vi "Spectrum Merge Wavelengths v10.5.0.vi"(2 "Wavelengths (nm)":dbl[](array[numeric]), 3 "Raw Spectrum":dbl[](array[numeric])) -> (0 "Spectrum-Array":dbl[][](array[numeric]), 1 "Spectrum-Cluster":T1(array[cluster]))   [LabVIEW 2010]
panel:
  out "Ausgangs-Cluster":T2
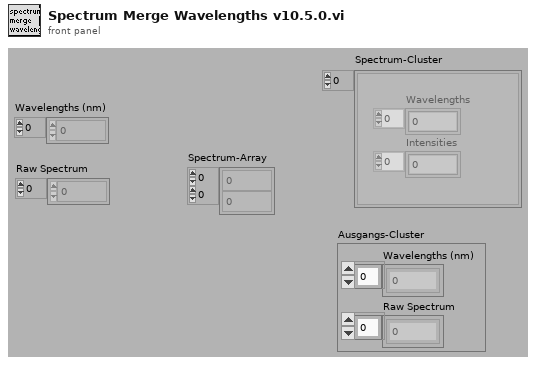
[diagram p1: front panel]
types:
  T1 = cluster{"Intensities":dbl[], "Wavelengths":dbl[]}[]
  T2 = cluster{"Wavelengths (nm)":dbl[], "Raw Spectrum":dbl[]}
  T3 = cluster{"Wavelengths (nm)":dbl[], "Raw Spectrum":dbl[]}[]
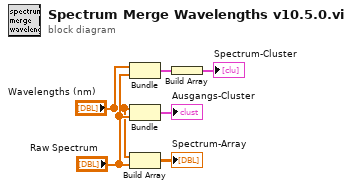
[diagram p0: block diagram]
diagram:
  n1 = Bundle("Wavelengths (nm)"="Wavelengths (nm)", "Raw Spectrum"="Raw Spectrum") -> (w4:T2)  [unwired: 1 in]
  n2 = Bundle("Wavelengths (nm)"="Wavelengths (nm)", "Raw Spectrum"="Raw Spectrum") -> (→"Ausgangs-Cluster":T2)  [unwired: 1 in]
  n3 = Build Array("Wavelengths (nm)", "Raw Spectrum") -> (→"Spectrum-Array":dbl[][])
  n4 = Build Array(w4) -> (→"Spectrum-Cluster":T3)
